vi "Result_Test.vi"(8 "error in (no error)":errorcluster caption="entrée d'erreur (pas d'erreur)", 11 "Delay en entrée":refnum<class "P2056_Get_IMEI.lvclass">) -> (0 "error out":errorcluster caption="sortie d'erreur", 3 "Delay en sortie":refnum<class "P2056_Get_IMEI.lvclass">)   [LabVIEW 2020, in "Library Test.lvlib" / "P2056_Get_IMEI.lvclass"]
uses:
  P2056_Get_IMEI.lvclass
  C:/Users/ngarcin/OneDrive - Altyor/Standard TB/Class/Test/Test (Default)/Test (Default).lvclass
  Test_Without_Instr/Test_Without_Inst.lvclass
  P2056_Get_IMEI.lvclass/P2056_Get_IMEI.ctl
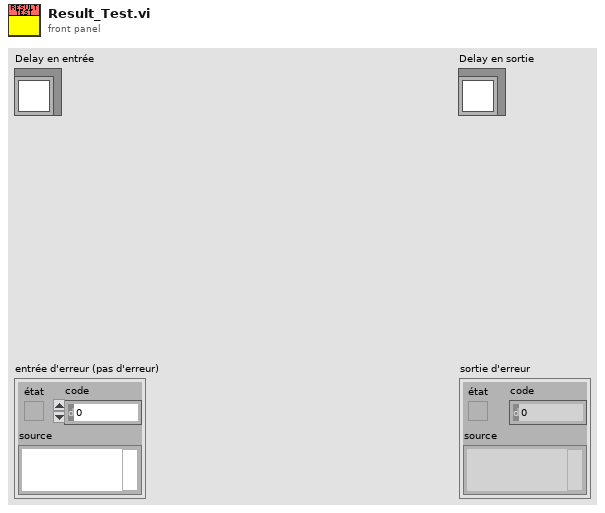
[diagram p1: front panel]
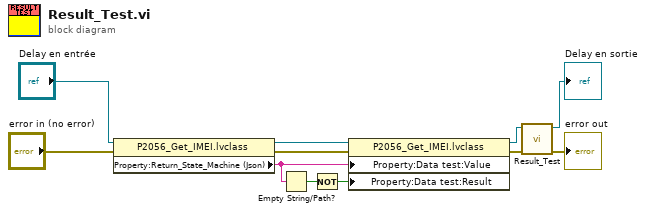
[diagram p0: block diagram]
diagram:
  n1 = property class="P2056_Get_IMEI.lvclass"(reference="Delay en entrée", error in="error in (no error)") -> (reference out=w9:refnum<class "P2056_Get_IMEI.lvclass">, error out=w8:errorcluster, "Property:Return_State_Machine (Json)"=w3:string)
  n2 = Empty String/Path?(string/path=w3) -> (empty?=w2:bool)
  n3 = Not(x=w2) -> (.not. x?=w1:bool)
  n4 = property class="P2056_Get_IMEI.lvclass"(reference=w9, error in=w8, "Property:Data test:Value"=w3, "Property:Data test:Result"=w1) -> (reference out=w4:refnum<class "P2056_Get_IMEI.lvclass">, error out=w6:errorcluster)
  n5 = call-parent "Result_Test.vi"("error in (no error)"=w6, "Test_Without_Inst en entrée"=w4) -> ("error out"=→"error out":errorcluster, "Test_Without_Inst en sortie"=→"Delay en sortie":refnum<class "P2056_Get_IMEI.lvclass">)  [unwired: 8 in]
